vi "RTS Chamber Door Files.vi"(7 "System Number":T2="Select System", 8 "error in (no error)":errorcluster, 11 "Search File Path Input":path) -> (0 "error out":errorcluster, 2 "Output":T1, 3 "Search File Path Output":path)   [LabVIEW 2016]
uses:
  Type Definitions/RTS Select System Number.ctl
  Type Definitions/RTS Test Pattern.ctl
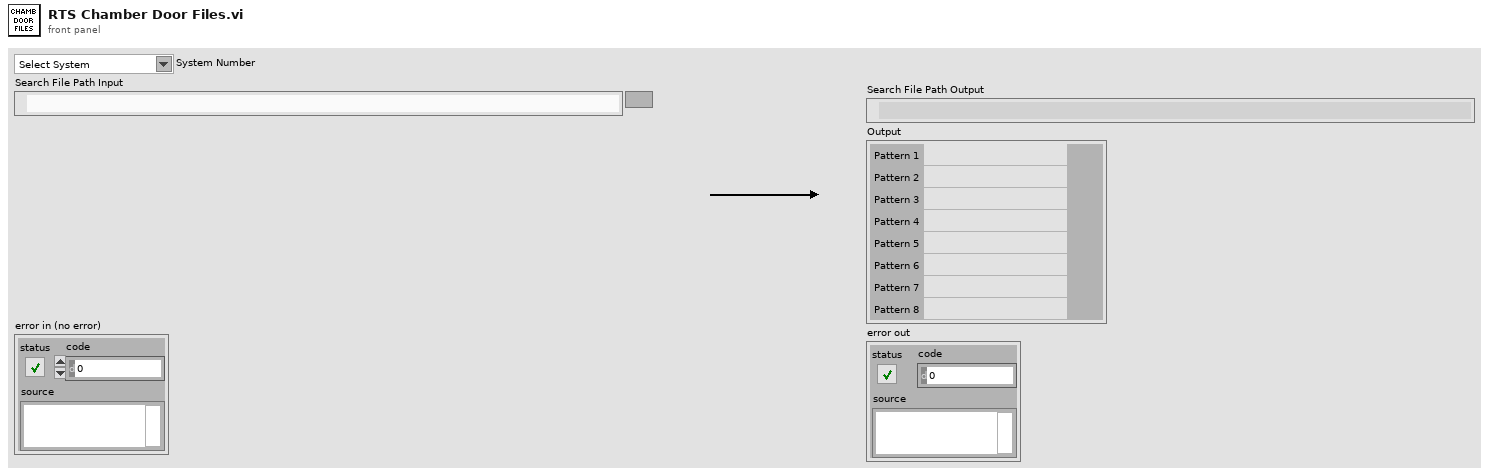
[diagram p1: front panel]
types:
  T1 = typedef "RTS Test Pattern.ctl" = cluster{" Pattern 1":path, "Pattern 2":path, "Pattern 3":path, "Pattern 4":path, "Pattern 5":path, "Pattern 6":path, "Pattern 7":path, "Pattern 8":path}
  T2 = typedef "RTS Select System Number.ctl" = string
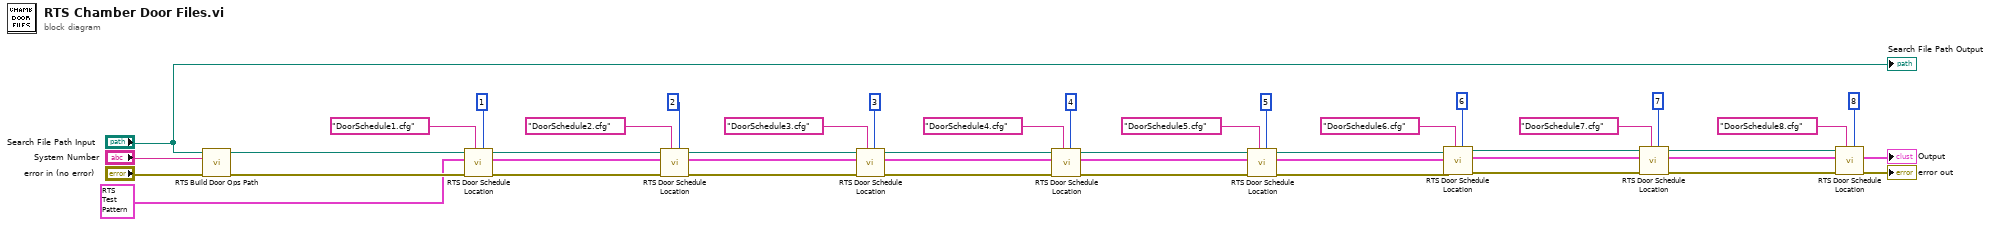
[diagram p0: block diagram]
diagram:
  n1 = call "RTS Build Door Ops Path.vi"("Error In"="error in (no error)", "System Number"="System Number", "Search File Path Input"="Search File Path Input") -> ("Error Out"=w10:errorcluster, "appended path"=w12:path)  [unwired: 7 in]
  n2 = call "RTS Door Schedule Location.vi"("Station"=u8 1, "File Name"="DoorSchedule1.cfg", "error in (no error)"=w10, "Input"=T1 {" Pattern 1"=path "", "Pattern 2"=path "", "Pattern 3"=path "", "Pattern 4"=path "", "Pattern 5"=path "", "Pattern 6"=path "", "Pattern 7"=path "", "Pattern 8"=path ""}, "Stripped Path Input"=w12) -> ("error out"=w16:errorcluster, "Output"=w9:T1, "Stripped Path Output"=w39:path)  [unwired: 4 in]
  n3 = call "RTS Door Schedule Location.vi"("Station"=u8 2, "File Name"="DoorSchedule2.cfg", "error in (no error)"=w16, "Input"=w9, "Stripped Path Input"=w39) -> ("error out"=w17:errorcluster, "Output"=w8:T1, "Stripped Path Output"=w40:path)  [unwired: 4 in]
  n4 = call "RTS Door Schedule Location.vi"("Station"=u8 3, "File Name"="DoorSchedule3.cfg", "error in (no error)"=w17, "Input"=w8, "Stripped Path Input"=w40) -> ("error out"=w18:errorcluster, "Output"=w7:T1, "Stripped Path Output"=w41:path)  [unwired: 4 in]
  n5 = call "RTS Door Schedule Location.vi"("Station"=u8 4, "File Name"="DoorSchedule4.cfg", "error in (no error)"=w18, "Input"=w7, "Stripped Path Input"=w41) -> ("error out"=w19:errorcluster, "Output"=w6:T1, "Stripped Path Output"=w42:path)  [unwired: 4 in]
  n6 = call "RTS Door Schedule Location.vi"("Station"=u8 5, "File Name"="DoorSchedule5.cfg", "error in (no error)"=w19, "Input"=w6, "Stripped Path Input"=w42) -> ("error out"=w20:errorcluster, "Output"=w5:T1, "Stripped Path Output"=w43:path)  [unwired: 4 in]
  n7 = call "RTS Door Schedule Location.vi"("Station"=u8 6, "File Name"="DoorSchedule6.cfg", "error in (no error)"=w20, "Input"=w5, "Stripped Path Input"=w43) -> ("error out"=w21:errorcluster, "Output"=w4:T1, "Stripped Path Output"=w44:path)  [unwired: 4 in]
  n8 = call "RTS Door Schedule Location.vi"("Station"=u8 7, "File Name"="DoorSchedule7.cfg", "error in (no error)"=w21, "Input"=w4, "Stripped Path Input"=w44) -> ("error out"=w22:errorcluster, "Output"=w3:T1, "Stripped Path Output"=w45:path)  [unwired: 4 in]
  n9 = call "RTS Door Schedule Location.vi"("Station"=u8 8, "File Name"="DoorSchedule8.cfg", "error in (no error)"=w22, "Input"=w3, "Stripped Path Input"=w45) -> ("error out"=→"error out":errorcluster, "Output"=→"Output":T1)  [unwired: 4 in, 1 out]
  "Search File Path Output" <- "Search File Path Input"
